vi "Query Power Sensor Zeroing Status.vi"(8 "error in (no error)":errorcluster, 10 "Instance (1)":i32=1 format="%.0g", 11 "VISA resource name":refnum<visa-resource-name>) -> (0 "error out":errorcluster, 2 "Reliability":i32, 3 "VISA resource name out":refnum<visa-resource-name>, 4 "Zeroing Status":bool)   [LabVIEW 2015, in "Rohde&Schwarz CMXP GPRF.lvlib"]
doc: "Starts a new single shot measurement and returns the results.\n\nAttribute:\nRSCMXPGPRF_ATTR_QUERY_SENSOR_MEASUREMENT_ZEROING\n\nRemote-control command:\nCALibration:GPRF:MEAS<i>:EPSensor:ZEROing?"
uses:
  <instrlib>/Rohde&Schwarz CMXP GPRF/Rohde&Schwarz CMXP GPRF.lvlib
  <instrlib>/Rohde&Schwarz CMXP GPRF/Private/rsidr_core.llb/rsidr_core.lvlib
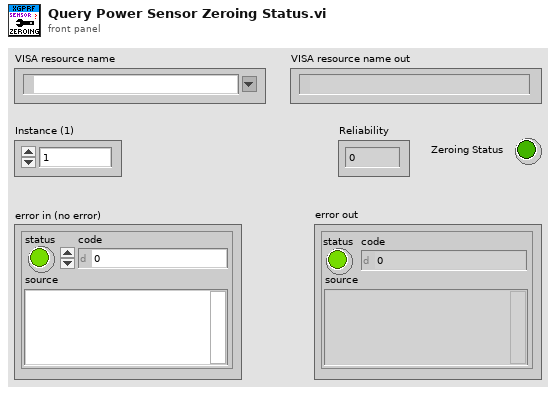
[diagram p1: front panel]
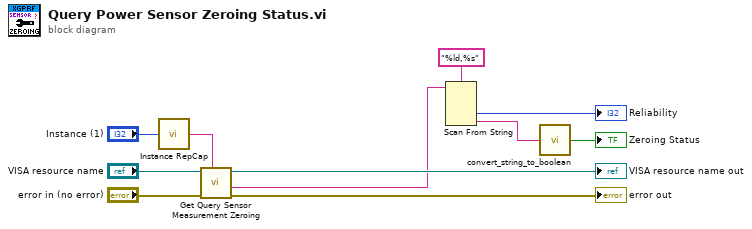
[diagram p0: block diagram]
diagram:
  n1 = call <instrlib>:"Instance RepCap.vi"("instance  in"="Instance (1)") -> ("instance out"=w5:string)
  n2 = call "Get Query Sensor Measurement Zeroing"("Repeated Capabilities"=w5, "error in (no error)"="error in (no error)", "instrument handle"="VISA resource name") -> ("error out"=→"error out":errorcluster, "Query Sensor Measurement Zeroing"=w1:string, "instrument handle out"=→"VISA resource name out":refnum<visa-resource-name>)  [unwired: 6 in]
  n3 = Scan From String(format string="%ld,%s", input string=w1) -> (output 1=→"Reliability":i32, output 2=w2:string)  [unwired: 4 in, 3 out]
  n4 = call <instrlib>:"convert_string_to_boolean.vi"("String in"=w2) -> ("boolean value out"=→"Zeroing Status":bool)  [unwired: 4 in]
